vi "AttackTacticVSS.vi"(6 "State":enum16{"Exit", "GoToBall", "BallToGoal"}(ring), 8 "First call?":bool=TRUE, 9 "Game in":refnum<class "Game.lvclass">, 10 "Robot":refnum<class "Robot.lvclass">, 11 "AttackTacticVSS in":refnum<class "AttackTacticVSS.lvclass">) -> (0 "error out 2":errorcluster, 2 "Robot out":refnum<class "Robot.lvclass">, 3 "AttackTacticVSS out":refnum<class "AttackTacticVSS.lvclass">)   [LabVIEW 2020, in "AttackTacticVSS.lvclass"]
uses:
  AttackTacticVSS.lvclass
  C:/Users/lucio/Desktop/Horie/ROBOIME/VSS_AI/Tactic_class/Tactic.lvclass
  Robot_class/Robot.lvclass
  Game_class/Game.lvclass
  Robot_class/tactics.ctl
  Tactic_class/Tactic.lvclass/Tactic.ctl
  Robot_class/Robot.lvclass/Robot.ctl
  Game_class/Read BallRef.vi
  Tactic_class/Read Skillbook.vi
  Robot_class/Write tactic.vi
  Skillbook_class/Skillbook.lvclass
  KickSkillVSS_class/KickSkillVSS.lvclass
  PenaltyPosSkillVSS_class/PenaltyPosSkillVSS.lvclass
  BallDispPosSkillVSS_class/BallDispPosSkillVSS.lvclass
  BallToGoalSkillVSS_class/BallToGoalSkillVSS.lvclass
  GoToBallSkillVSS_class/GoToBallSkillVSS.lvclass
  DefBallPosSkillVSS_class/DefBallPosSkillVSS.lvclass
  HaltSkill_class/HaltSkill.lvclass
  KeeperDefPosSkillVSS_class/KeeperDefPosSkillVSS.lvclass
  GoToBallKeeperSkillVSS_class/GoToBallKeeperSkillVSS.lvclass
  RotateWallSkillVSS_class/RotateWallSkillVSS.lvclass
  Ball_class/Ball.lvclass
panel:
  out "x .or. y?":bool
  in  "error in (no error) 2":errorcluster
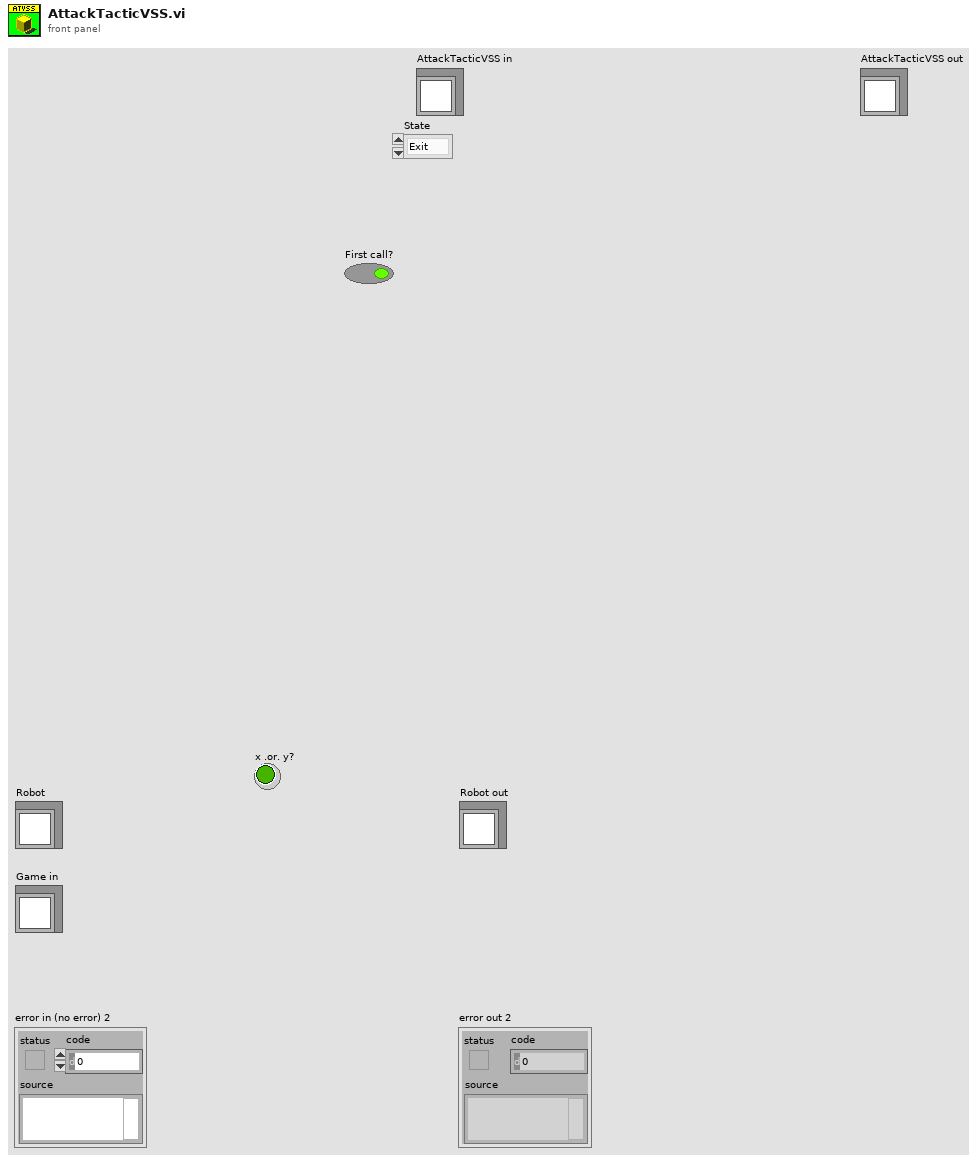
[diagram p1: front panel]
types:
  T1 = typedef "tactics.ctl" = enum16{"ReceivePassInFuturePoint", "Roller", "PrepareRollToPassRollerGoTo", "PrepareRollToPassReceiverGoTo", "WaitRoll", "PositionToRoll", "PenaltyAttacker", "PassObserver", "PenaltyDefense", "TableReceiverTactic", "Test", "DefendGoal", "Marker", "FollowAttacker", "DefendArea", "Shoot", "AttackerAimGoal", "AttackerBallOutOfField", "AttackerBlock", "AttackerStop", "Duelist", "Halt", "ZigZag", "GoTo", "Timeout", "KickToPassReceiver", "PositionToReceivePass", "DefendAreaVSS", "DefendGoalVSS", "KickVSS", "AttackVSS", "DispBallVSS", "PenaltyAttackVSS", "WaitPass"}
  T2 = cluster{"KickSkillVSS":refnum<class "KickSkillVSS.lvclass">, "PenaltyPosSkillVSS":refnum<class "PenaltyPosSkillVSS.lvclass">, "BallDispPosSkillVSS":refnum<class "BallDispPosSkillVSS.lvclass">, "BallToGoalSkillVSS":refnum<class "BallToGoalSkillVSS.lvclass">, "GoToBallSkillVSS":refnum<class "GoToBallSkillVSS.lvclass">, "DefBallPosSkillVSS":refnum<class "DefBallPosSkillVSS.lvclass">, "HaltSkill":refnum<class "HaltSkill.lvclass">, "KeeperDefPosSkillVSS":refnum<class "KeeperDefPosSkillVSS.lvclass">, "GoToBallKeeperSkillVSS":refnum<class "GoToBallKeeperSkillVSS.lvclass">, "RotateWallSkillVSS":refnum<class "RotateWallSkillVSS.lvclass">}
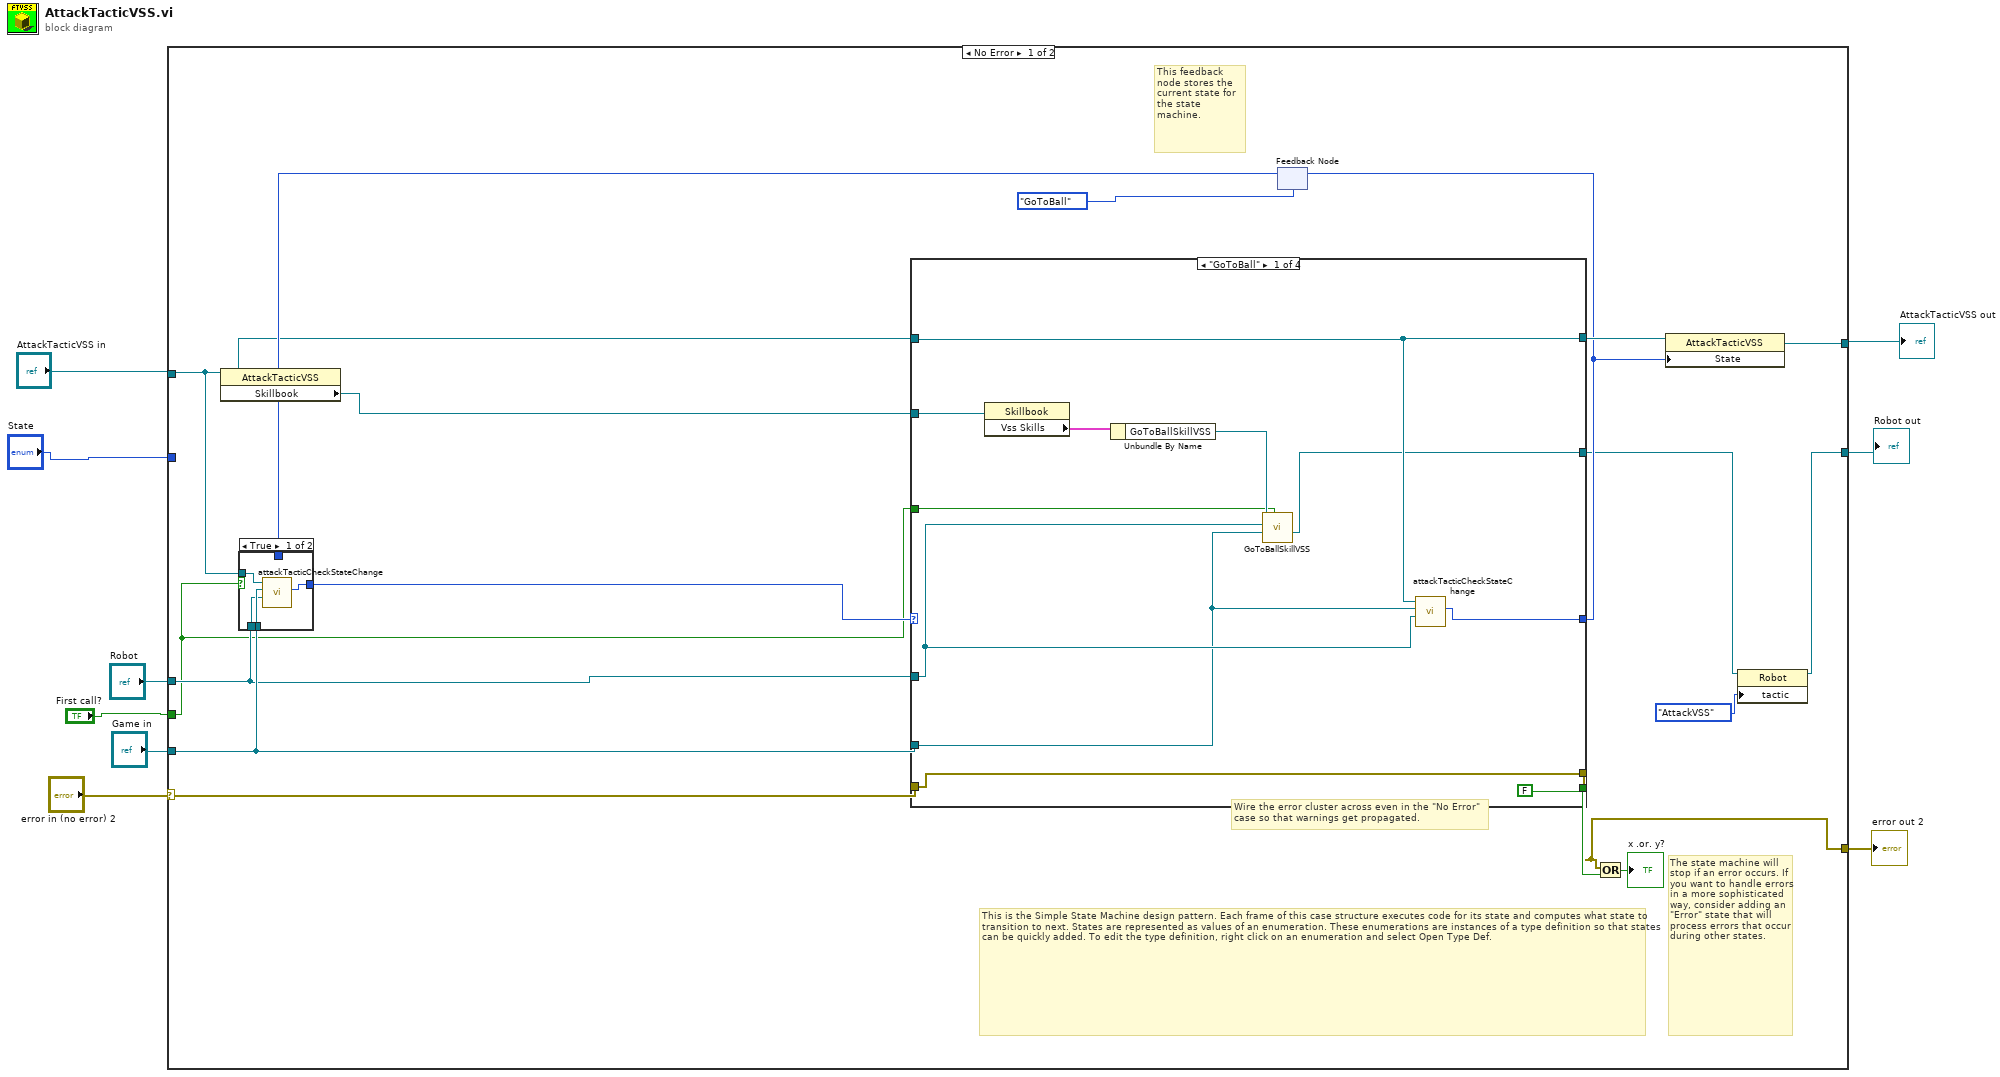
[diagram p0: block diagram]
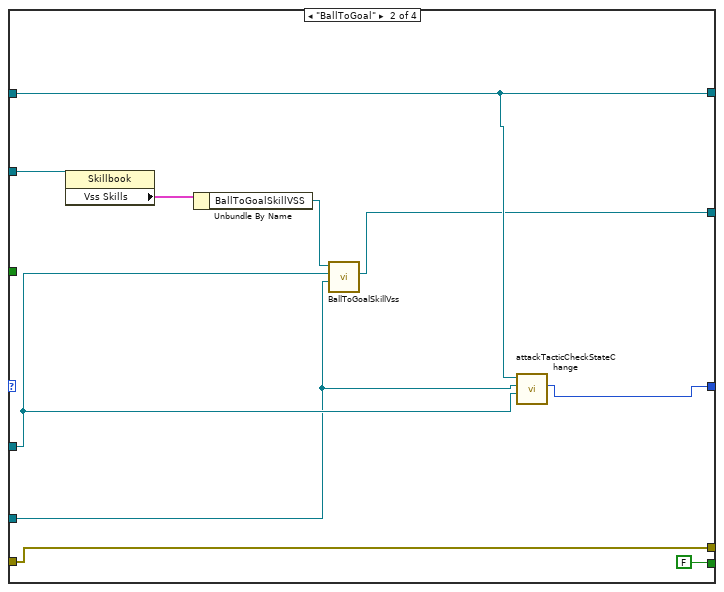
[diagram p3: hidden frame]
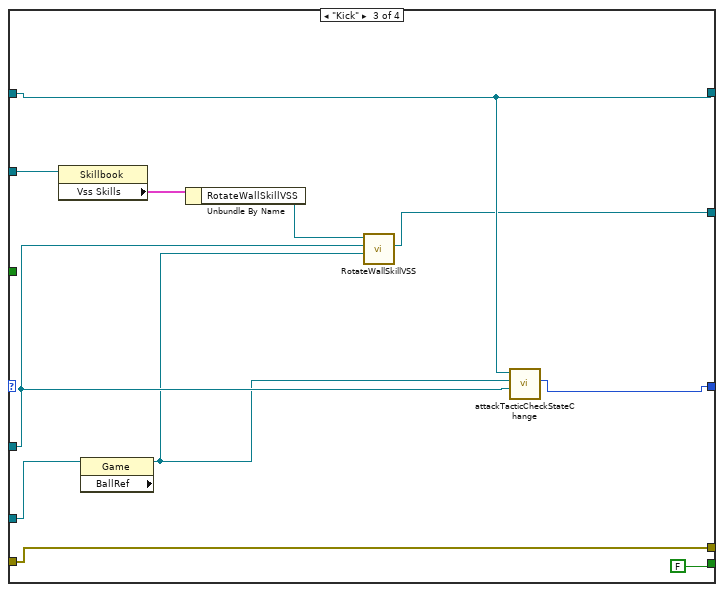
[diagram p4: hidden frame]
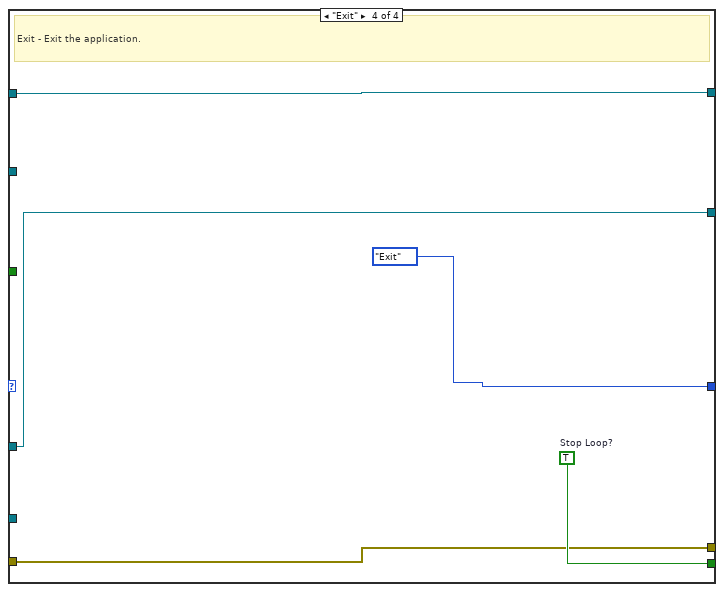
[diagram p5: hidden frame]
diagram:
  n1 = case shown="No Error" "error in (no error) 2" {
    selector: "error in (no error) 2" -> [w23 w72]
    tunnel: [w22 w72] -> w8
    tunnel: [w20 w71] -> w3
    tunnel: "AttackTacticVSS in" -> [w13 w71]
    tunnel: "Robot" -> [w11 w70]
    tunnel: "Game in" -> [w12 _]
    tunnel: [w17 w70] -> w5
    tunnel: "State" -> [_ _]
    tunnel: "First call?" -> [w10 _]
    frame No Error {
      # "The state machine will stop if an error occurs. If you want to handle errors in a more sophisticated way, consider adding an \"Error\" state that will process errors that occur during other states."
      # "This feedback node stores the current state for the state machine."
      # "This is the Simple State Machine design pattern. Each frame of this case structure executes code for its state and computes what state to transition to next. States are represented as values of an enumeration. These enumerations are instances of a type definition so that states can be quickly added. To edit the type definition, right click on an enumeration and select Open Type Def."
      # "Wire the error cluster across even in the \"No Error\"\ncase so that warnings get propagated."
      n2 = property class="AttackTacticVSS"(reference=w13) -> ("Skillbook"=w25:refnum<class "Skillbook.lvclass">)  [unwired: 1 in, 2 out]
      n3 = feedback #1(enum16{"Kick", "Exit", "GoToBall", "BallToGoal"}."GoToBall" ("State")) -> (w16:enum16{"Kick", "Exit", "GoToBall", "BallToGoal"})
      n4 = case shown="True" w10 {
        tunnel: [w31 w32] -> w15
        tunnel: w16 -> [_ w32]
        tunnel: w13 -> [w30 _]
        tunnel: w12 -> [w29 _]
        tunnel: w11 -> [w28 _]
        frame True {
          n5 = call "attackTacticCheckStateChange.vi"("Robot In"=w28, "Game in"=w29, "AttackTacticVSS in"=w30) -> ("State"=w31:enum16{"Kick", "Exit", "GoToBall", "BallToGoal"})  [unwired: 6 in, 2 out]
        }
        frame False {
        }
      }
      n6 = case shown="\"GoToBall\"" w15 {
        tunnel: [w41 w50 w61 enum16{"Kick", "Exit", "GoToBall", "BallToGoal"}."Exit" ("State")] -> w21
        tunnel: [FALSE FALSE FALSE w69] -> w27
        tunnel: w25 -> [w42 w52 w63 _]
        tunnel: w11 -> [w35 w45 w57 w68]
        tunnel: [w36 w46 w54 w68] -> w18
        tunnel: [w40 w51 w62 w67] -> w24
        tunnel: w13 -> [w40 w51 w62 w67]
        tunnel: w12 -> [w34 w44 w58 _]
        tunnel: [w39 w49 w59 w66] -> w22
        tunnel: w23 -> [w39 w49 w59 w66]
        tunnel: w10 -> [w33 _ _ _]
        frame "GoToBall" {
          n7 = property class="Skillbook"(reference=w42) -> ("Vss Skills"=w43:T2)  [unwired: 1 in, 2 out]
          n8 = Unbundle By Name(w43) -> ("GoToBallSkillVSS"=w37:refnum<class "GoToBallSkillVSS.lvclass">)
          n9 = call "GoToBallSkillVSS.vi"("First call?"=w33, "Game"=w34, "Robot in"=w35, "GoToBallSkillVSS in"=w37) -> ("Robot out"=w36:refnum<class "Robot.lvclass">)  [unwired: 5 in, 2 out]
          n10 = call "attackTacticCheckStateChange.vi"("Robot In"=w35, "Game in"=w34, "AttackTacticVSS in"=w40) -> ("State"=w41:enum16{"Kick", "Exit", "GoToBall", "BallToGoal"})  [unwired: 6 in, 2 out]
        }
        frame "BallToGoal" {
          n11 = property class="Skillbook"(reference=w52) -> ("Vss Skills"=w53:T2)  [unwired: 1 in, 2 out]
          n12 = Unbundle By Name(w53) -> ("BallToGoalSkillVSS"=w47:refnum<class "BallToGoalSkillVSS.lvclass">)
          n13 = call "BallToGoalSkillVss.vi"("Game"=w44, "Robot in"=w45, "BallToGoalSkillVSS in"=w47) -> ("Robot out"=w46:refnum<class "Robot.lvclass">)  [unwired: 6 in, 2 out]
          n14 = call "attackTacticCheckStateChange.vi"("Robot In"=w45, "Game in"=w44, "AttackTacticVSS in"=w51) -> ("State"=w50:enum16{"Kick", "Exit", "GoToBall", "BallToGoal"})  [unwired: 6 in, 2 out]
        }
        frame "Kick" {
          n15 = property class="Skillbook"(reference=w63) -> ("Vss Skills"=w64:T2)  [unwired: 1 in, 2 out]
          n16 = property class="Game" props=["BallRef"](reference=w58) -> (reference out=w55:refnum<class "Game.lvclass">)  [unwired: 1 in, 2 out]
          n17 = Unbundle By Name(w64) -> ("RotateWallSkillVSS"=w56:refnum<class "RotateWallSkillVSS.lvclass">)
          n18 = call "RotateWallSkillVSS.vi"("Game"=w55, "Robot"=w57, "RotateWallSkillVSS in"=w56) -> ("Robot out"=w54:refnum<class "Robot.lvclass">)  [unwired: 6 in, 2 out]
          n19 = call "attackTacticCheckStateChange.vi"("Robot In"=w57, "Game in"=w55, "AttackTacticVSS in"=w62) -> ("State"=w61:enum16{"Kick", "Exit", "GoToBall", "BallToGoal"})  [unwired: 6 in, 2 out]
        }
        frame "Exit" {
          w69 = TRUE  # Stop Loop?
          # "Exit - Exit the application."
        }
      }
      n20 = feedback-in #1(w21) -> ()
      n21 = Or(x=w22, y=w27) -> (x .or. y?=→"x .or. y?":bool)
      n22 = property class="AttackTacticVSS"(reference=w24, "State"=w21) -> (reference out=w20:refnum<class "AttackTacticVSS.lvclass">)  [unwired: 1 in, 1 out]
      n23 = property class="Robot"(reference=w18, "tactic"=tactics."AttackVSS") -> (reference out=w17:refnum<class "Robot.lvclass">)  [unwired: 1 in, 1 out]
    }
    frame Error {
    }
  }
  "AttackTacticVSS out" <- w3
  "error out 2" <- w8
  "Robot out" <- w5
